vi "Send Create Process.vi"(6 "Database":T1, 7 "Message Priority (Normal)":T2=enum."Normal", 8 "error in (no error)":errorcluster, 9 "Run?":bool=TRUE, 10 "Process Name":string, 11 "Message Enqueuer":refnum<class "Message Enqueuer.lvclass">) -> (0 "error out":errorcluster, 3 "Message Enqueuer out":refnum<class "Message Enqueuer.lvclass">)   [LabVIEW 2016, in "CS++DSCManager.lvlib" / "Create Process Msg.lvclass"]
doc: "Sends the <B>CS++DSCManager.lvlib:Create Process Msg.lvclass</B> message.\n\n<B>CS++DSCManager.lvlib:CS++DSCManager.lvclass:Create Process.vi</B> Description:\n\nCreates an empty process in the Shared Variable Engine (SVE) on the host computer. The process that you want to create replaces an existing process if the two processes have the same name."
uses:
  Create Process Msg.lvclass
  <vilib>/ActorFramework/Message Enqueuer/Message Enqueuer.lvclass
  <vilib>/ActorFramework/Message Enqueuer/Message Priority.ctl
  C:/Program Files (x86)/National Instruments/LabVIEW 2016/vi.lib/ActorFramework/Message/Message.lvclass
  Create Process Msg.lvclass/Create Process Msg.ctl
  <vilib>/ActorFramework/Message Enqueuer/Message Enqueuer.lvclass/Message Enqueuer.ctl
  <vilib>/ActorFramework/Message Priority Queue/Priority Enqueue.vi
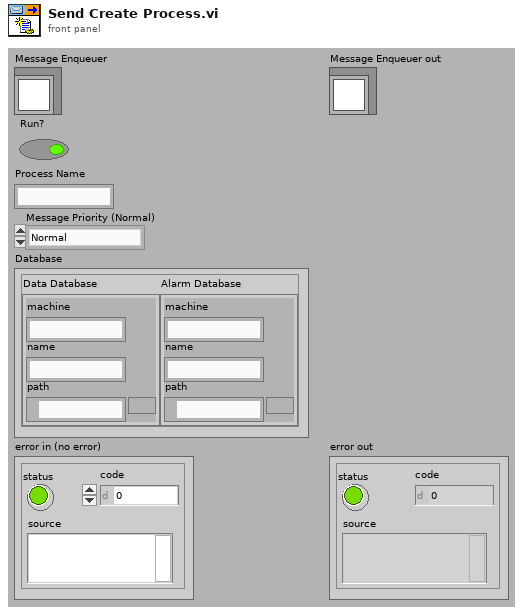
[diagram p1: front panel]
types:
  T1 = cluster{"Data Database":cluster{"machine":string, "name":string, "path":path}, "Alarm Database":cluster{"machine":string, "name":string, "path":path}}
  T2 = typedef "Actor Framework.lvlib/Message Enqueuer.lvclass/Message Priority.ctl" = enum16{"Low", "Normal", "High"}
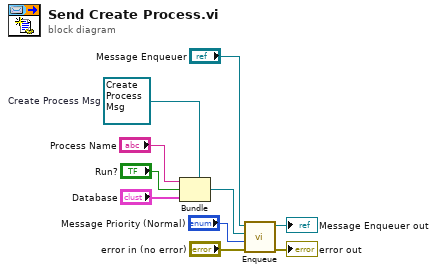
[diagram p0: block diagram]
diagram:
  w4 = refnum<class "Create Process Msg.lvclass"> refnum  # Create Process Msg
  n1 = Bundle(cluster=w4, "Process Name", "Run?", "Database") -> (w7:refnum<class "Create Process Msg.lvclass">)
  n2 = call <vilib>:"Enqueue.vi"("error in (no error)"="error in (no error)", "Message Priority (Normal)"="Message Priority (Normal)", "Message"=w7, "Message Enqueuer in"="Message Enqueuer") -> ("error out"=→"error out":errorcluster, "Message Enqueuer out"=→"Message Enqueuer out":refnum<class "Message Enqueuer.lvclass">)  [unwired: 6 in]
